vi "Restart.LocalStop.Read.vi"(8 "error in (no error)":errorcluster, 11 "Data Value Reference in":refnum<data-value>) -> (0 "error out":errorcluster, 3 "LocalStop":bool)   [LabVIEW 2019, in "Diagnostics Addon Engine.lvlib"]
uses:
  Diagnostics Addon Engine.lvlib
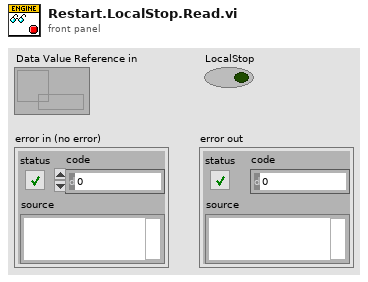
[diagram p1: front panel]
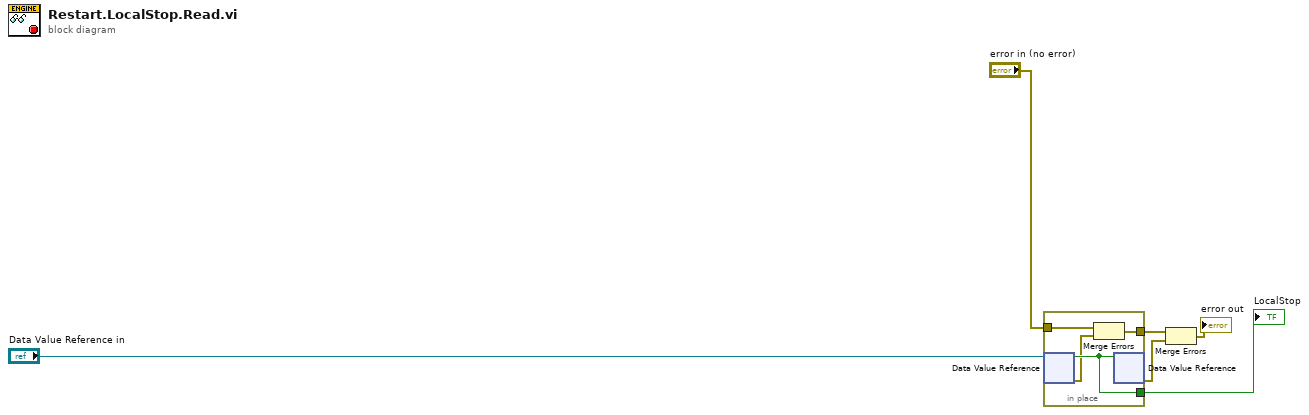
[diagram p0: block diagram]
diagram:
  n1 = in-place {
    in-place-border: [w10] -> w6
    in-place-border: "error in (no error)" -> [w9]
    in-place-border: [w7] -> w3
    n2 = in-place-dvr #1("Data Value Reference in") -> (w10:bool, w8:errorcluster)
    n3 = Merge Errors(w9, w8) -> (w7:errorcluster)
    n4 = in-place-dvr #1(w10) -> (w4:errorcluster)  [unwired: 1 out]
  }
  "LocalStop" <- w6
  n5 = Merge Errors(w3, w4) -> (→"error out":errorcluster)
